vi "Configure PLL Mode.vi"(8 "error in (no error)":errorcluster, 10 "PLL Mode":T1, 11 "MXA in":refnum<class "MXA.lvclass">) -> (0 "error out":errorcluster, 3 "MXA out":refnum<class "MXA.lvclass">)   [LabVIEW 2020, in "MXA.lvclass"]
uses:
  MXA.lvclass
  C:/Sandbox/Git_Sandbox/WiSpry Test Framework source code (LV20)/WiSpry Test Framework/Instruments/Instrument.lvclass
  Controls/PLL Mode.ctl
  Instrument.lvclass
  Spectrum Analyzer.lvclass
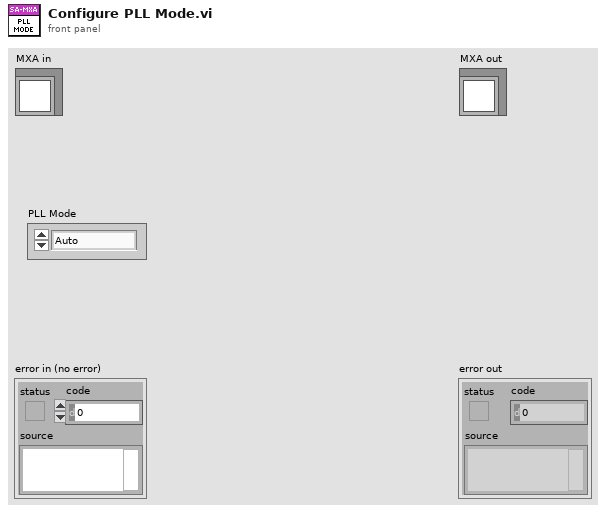
[diagram p1: front panel]
types:
  T1 = typedef "Spectrum Analyzer.lvclass/PLL Mode.ctl" = enum16{"Auto", "Narrow", "Normal", "Wide"}
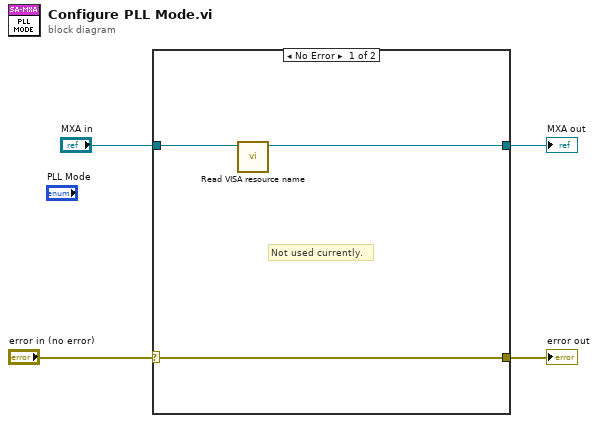
[diagram p0: block diagram]
diagram:
  n1 = case shown="No Error" "error in (no error)" {
    selector: "error in (no error)" -> [w5 w9]
    tunnel: "MXA in" -> [w7 w8]
    tunnel: [w5 w9] -> w4
    tunnel: [w6 w8] -> w1
    frame No Error {
      # "Not used currently."
      n2 = call "Read VISA resource name.vi"("Instrument in"=w7) -> ("Instrument out"=w6:refnum<class "MXA.lvclass">)  [unwired: 9 in, 1 out]
    }
    frame Error {
    }
  }
  "error out" <- w4
  "MXA out" <- w1
